vi "TimeBasedDrive.vi"(10 "Time (ms)":u32, 11 "Motor Value":dbl) -> ()   [LabVIEW 2012]
uses:
  Robot Global Data.vi
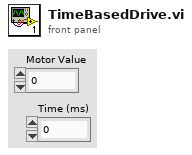
[diagram p1: front panel]
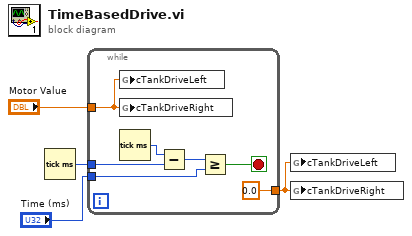
[diagram p0: block diagram]
diagram:
  n1 = Tick Count (ms)() -> (millisecond timer value=w2:u32)
  n2 = while {
    tunnel: "Time (ms)" -> [w8]
    tunnel: "Motor Value" -> [w6]
    tunnel: w2 -> [w10]
    tunnel: [0.0] -> w1
    stop <- w7 stop-if-true
    n3 = global write "Robot Global Data.vi" "cTankDriveLeft"(w6) -> ()
    n4 = global write "Robot Global Data.vi" "cTankDriveRight"(w6) -> ()
    n5 = Tick Count (ms)() -> (millisecond timer value=w11:u32)
    n6 = Subtract(x=w11, y=w10) -> (x-y=w9:u32)
    n7 = Greater Or Equal?(x=w9, y=w8) -> (x >= y?=w7:bool)
  }
  n8 = global write "Robot Global Data.vi" "cTankDriveLeft"(w1) -> ()
  n9 = global write "Robot Global Data.vi" "cTankDriveRight"(w1) -> ()
